vi "sv_Waterfall for Octave Global.vi"() -> ()   [LabVIEW 2017]
panel:
  in  "axis labels":T1
  in  "frontmost (T)":bool=TRUE
  in  "bandedge freq. list":T2(array[cluster]) {"midband" format="%.2f"; "f high" format="%.2f"; "f low" format="%.2f"}
  in  "display  size":cluster{"width":u32, "heigth":u32}={"width"=400, "heigth"=300}
  in  "occurrence":refnum<k4>
  in  "colors":T3={"frame"=16763904, "plot"=52224, "background"=0}
  in  "autoscale (T)":bool=TRUE
  in  "baseline":dbl format="%.2f"
  in  "set baseline (F)":bool
  in  "clear graph before redrawing (F)":bool
  in  "y0 and delta y":cluster{"y0":dbl, "delta y":dbl}={"y0"=0.0, "delta y"=1.0} {"delta y" format="%.2f"; "y0" format="%.2f"}
  in  "waterfall data":dbl[][](array[numeric]) format="%.2f"
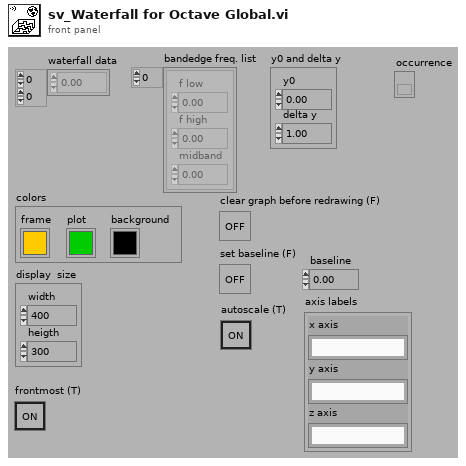
[diagram p1: front panel]
types:
  T1 = cluster{"x axis":string, "y axis":string, "z axis":string}
  T2 = cluster{"f low":dbl, "f high":dbl, "midband":dbl}[]
  T3 = cluster{"frame":u32, "plot":u32, "background":u32}
diagram:
